vi "process_api_vi_ref.vi"   [LabVIEW 2015]
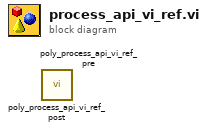
[diagram p0: block diagram]
diagram:
  n1 = call "poly_process_api_vi_ref_post.vi"() -> ()  [unwired: 10 in, 2 out]
  n2 = call "poly_process_api_vi_ref_pre.vi"() -> ()  [unwired: 10 in, 2 out]
